vi "etc_XCITE_OpenDeviceEx.vi"(8 "error in (no error)":errorcluster {"code" format="%x"}, 11 "h":u64) -> (0 "error out":errorcluster {"code" format="%x"}, 2 "ErrorMessage":i32 format="%x", 3 "h out":u64)   [LabVIEW 2019, in "XCite.lvlib"]
doc: "Opens communication with the slelected X-cite device."
uses:
  XCite.lvlib
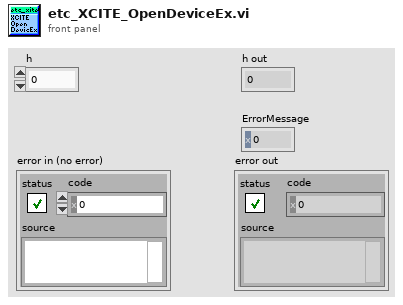
[diagram p1: front panel]
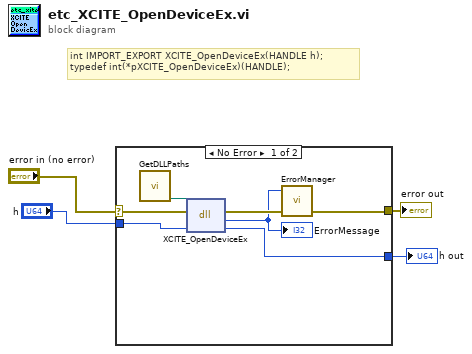
[diagram p0: block diagram]
diagram:
  # "int IMPORT_EXPORT XCITE_OpenDeviceEx(HANDLE h);\ntypedef int(*pXCITE_OpenDeviceEx)(HANDLE);"
  n1 = case shown="No Error" "error in (no error)" {
    selector: "error in (no error)" -> [w11 w13]
    tunnel: [w9 w13] -> w4
    tunnel: "h" -> [w7 w12]
    tunnel: [w6 w12] -> w2
    frame No Error {
      n2 = call "GetDLLPaths.vi"() -> ("etc_xcite_path"=w5:path)  [unwired: 8 in, 3 out]
      n3 = dll-call lib="C:/LabVIEWDevFall2024/pco.labview/labview_sdk/runtime/bin64/etc_xcite.dll" fn="XCITE_OpenDeviceEx"(path in=w5, error in=w11, "h"=w7) -> (error out=w10:errorcluster, "return type"=w8:i32, "h"=w6:u64)  [unwired: 1 in, 1 out]
      "ErrorMessage" <- w8
      n4 = call "ErrorManager.vi"("error in (no error)"=w10, "error code"=w8) -> ("error out"=w9:errorcluster)  [unwired: 2 in, 1 out]
    }
    frame Error {
    }
  }
  "error out" <- w4
  "h out" <- w2
